vi "setConfigVals.vi"(8 "file path":path) -> (0 "Axial inc (mm)":dbl, 1 "zPosInit (mm)":dbl, 2 "yPosInit (mm)":dbl, 3 "xPosFin (mm)":dbl, 4 "yPosFin (mm)":dbl, 5 "xPosInit (mm)":dbl, 6 "zPosFin (mm)":dbl, 7 "Lateral inc (mm)":dbl)   [LabVIEW 2015]
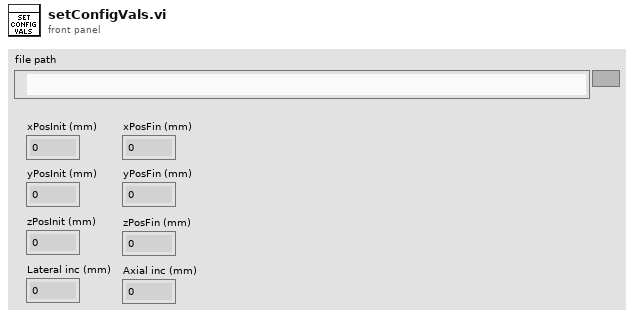
[diagram p1: front panel]
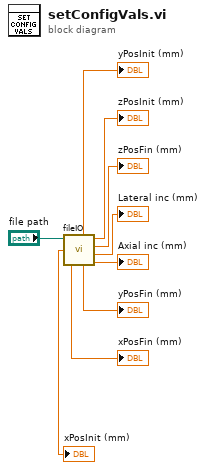
[diagram p0: block diagram]
diagram:
  n1 = call "fileIO.vi"("file path (dialog if empty)"="file path") -> ("Axial inc (mm)"=→"Axial inc (mm)":dbl, "yPosFin (mm)"=→"yPosFin (mm)":dbl, "Lateral inc (mm)"=→"Lateral inc (mm)":dbl, "zPosFin (mm)"=→"zPosFin (mm)":dbl, "yPosInit (mm)"=→"yPosInit (mm)":dbl, "zPosInit (mm)"=→"zPosInit (mm)":dbl, "xPosFin (mm)"=→"xPosFin (mm)":dbl, "xPosInit (mm)"=→"xPosInit (mm)":dbl)
